vi "test read png with user info.vi"() -> ()   [LabVIEW 2014]
uses:
  POLARIS Vision utility.lvlib
panel:
  out "value":variant
  out "Image":T1(plugin-control)
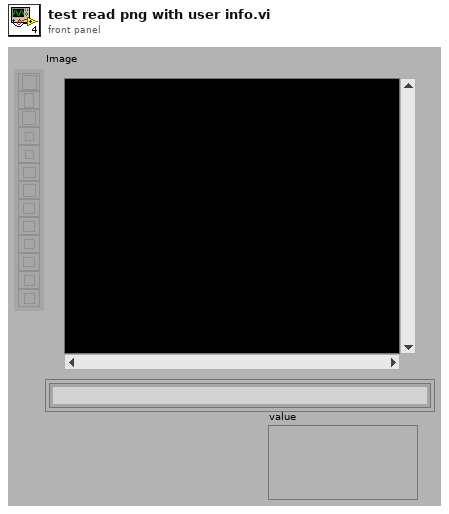
[diagram p1: front panel]
types:
  T1 = typedef "IMAQ Image.ctl" = refnum<image>
  T2 = cluster{"Name":string, "type string":i16[], "data string":string}
  T3 = typedef "Image Type" = u32
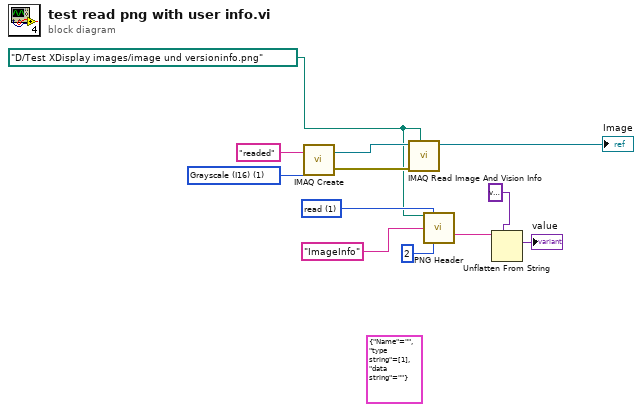
[diagram p0: block diagram]
diagram:
  (unwired) T2 {"Name"="", "type string"=[1], "data string"=""}
  w5 = path "D:/Test XDisplay images/image und versioninfo.png" ("File Path")
  w7 = u16 1 items=["Write", "read"] ("Mode")
  w12 = T3 1 items=["Grayscale (U8)", "Grayscale (I16)", "Grayscale (SGL)", "Complex (CSG)", "RGB (U32)", "HSL (U32)", "RGB (U64)", "Grayscale (U16)"] ("Image Type")
  n1 = call "IMAQ Create"("Image Name"="readed", "Image Type"=w12) -> ("New Image"=w10:T1, "error out"=w9:errorcluster)  [unwired: 3 in]
  n2 = call "IMAQ Read Image And Vision Info"("File Path"=w5, "error in (no error)"=w9, "Image"=w10) -> ("Image Out"=→"Image":T1)  [unwired: 6 in, 2 out]
  n3 = call "PNG Header.vi"("Path In"=w5, "Mode"=w7, "header in"="ImageInfo", "index (-1 last entry)"=2) -> ("string out"=w3:string)  [unwired: 7 in, 4 out]
  n4 = Unflatten From String(type=variant ("variant"), binary string=w3) -> (value=→"value":variant)  [unwired: 3 in, 2 out]
